vi "register child queue.vi"(8 "error in":errorcluster, 10 "queue":refnum<class "identifying queue.lvclass">, 11 "communicator in":refnum<class "communicator.lvclass">) -> (0 "error out":errorcluster, 3 "communicator out":refnum<class "communicator.lvclass">)   [LabVIEW 2015, in "communicator.lvclass"]
uses:
  communicator.lvclass
  communicator queue/identifying queue.lvclass
  communicator.lvclass/communicator.ctl
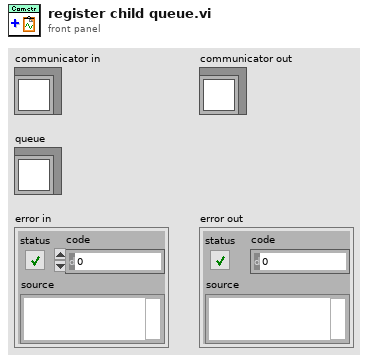
[diagram p1: front panel]
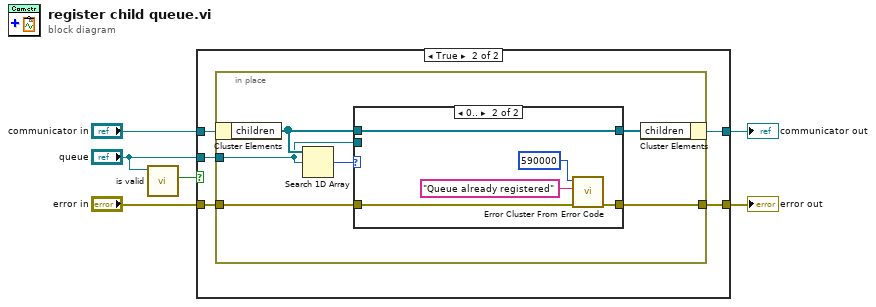
[diagram p0: block diagram]
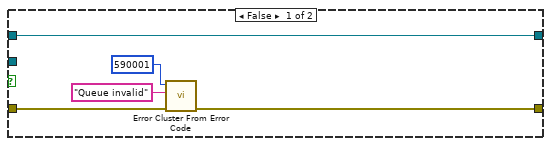
[diagram p2: hidden frame]
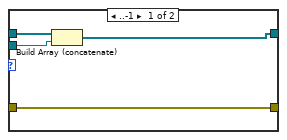
[diagram p3: hidden frame]
diagram:
  n1 = call "is valid.vi"("identifying queue in"="queue") -> ("valid?"=w6:bool)  [unwired: 9 in, 1 out]
  n2 = case shown="True" w6 {
    tunnel: "communicator in" -> [w11 w16]
    tunnel: [w11 w15] -> w3
    tunnel: [w9 w14] -> w4
    tunnel: "error in" -> [w10 w13]
    tunnel: "queue" -> [_ w12]
    frame False {
      n3 = call <vilib>:"Error Cluster From Error Code.vi"("error in (no error)"=w10, "error message (\"\")"="Queue invalid" ("error message (\"\")"), "error code (0)"=590001) -> ("error out"=w9:errorcluster)  [unwired: 6 in]
    }
    frame True {
      n4 = in-place {
        in-place-border: [w20] -> w14
        in-place-border: w13 -> [w21]
        in-place-border: w12 -> [w17]
        n5 = in-place-cluster #1(w16) -> ("children"=w18:refnum<class "identifying queue.lvclass">[])
        n6 = Search 1D Array(1D array=w18, element=w17) -> (index of element=w22:i32)  [unwired: 1 in]
        n7 = case shown="0.." w22 {
          tunnel: w21 -> [w26 w29]
          tunnel: [w26 w28] -> w20
          tunnel: [w23 w27] -> w19
          tunnel: w18 -> [w25 w27]
          tunnel: w17 -> [w24 _]
          frame ..-1 {
            n8 = Build Array (concatenate)(w25, w24) -> (w23:refnum<class "identifying queue.lvclass">[])
          }
          frame 0.. {
            n9 = call <vilib>:"Error Cluster From Error Code.vi"("error in (no error)"=w29, "error message (\"\")"="Queue already registered" ("error message (\"\")"), "error code (0)"=590000) -> ("error out"=w28:errorcluster)  [unwired: 6 in]
          }
        }
        n10 = in-place-cluster #1("children"=w19) -> (w15:refnum<class "communicator.lvclass">)
      }
    }
  }
  "error out" <- w4
  "communicator out" <- w3
